vi "Set Capillary Valve.vi"(8 "error in (no error)":errorcluster, 9 "Interlock Chain.lvclass":refnum<class "Interlock Chain.lvclass">, 10 "Open? (False)":bool, 11 "Capillary Line in":refnum<class "Capillary Line.lvclass">) -> (0 "error out":errorcluster, 3 "Capillary Line out":refnum<class "Capillary Line.lvclass">)   [LabVIEW 2015, in "cRIO-Carbondioxide.lvlib" / "CO2-Actor.lvlib" / "Capillary Line.lvclass"]
uses:
  Capillary Line.lvclass
  Interlocks/Interlock Chain/Interlock Chain.lvclass
  <vilib>/ActorFramework/Actor/Actor.lvclass/Actor.ctl
  <vilib>/ActorFramework/Message Enqueuer/Message Enqueuer.lvclass/Message Enqueuer.ctl
  Capillary Line.lvclass/Capillary Line.ctl
  Valve Messages/Write Bit Field Msg/Write Bit Field Msg.lvclass/Write Bit Field Msg.ctl
  <vilib>/ActorFramework/Actor/Read Self Enqueuer.vi
  <vilib>/ActorFramework/Message Enqueuer/Enqueue.vi
  <vilib>/ActorFramework/Message Enqueuer/Init from Existing Queue.vi
  <vilib>/ActorFramework/Message Priority Queue/Priority Enqueue.vi
  <vilib>/ActorFramework/Actor/Actor.lvclass
  <vilib>/ActorFramework/Message Enqueuer/Message Enqueuer.lvclass
  Valve Messages/Write Bit Field Msg/Write Bit Field Msg.lvclass
  CO2 Actor/CO2 Actor.lvclass
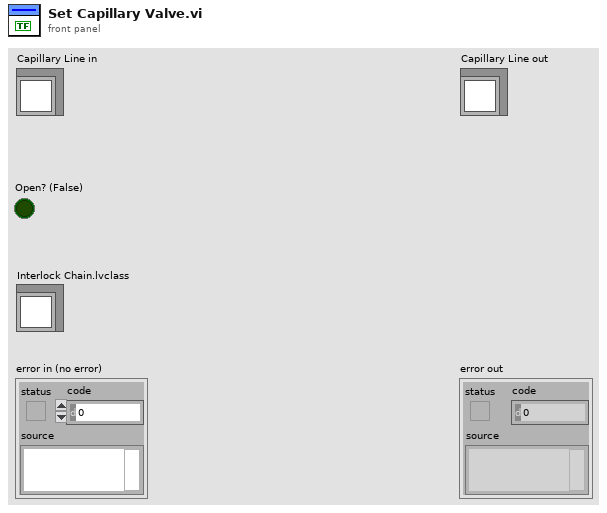
[diagram p1: front panel]
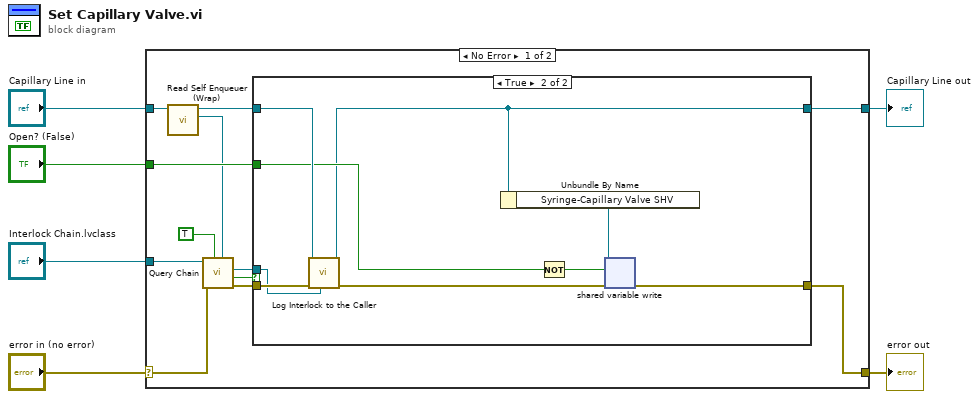
[diagram p0: block diagram]
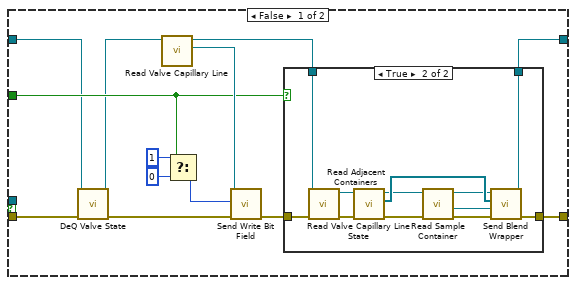
[diagram p2: hidden frame]
diagram:
  n1 = case shown="No Error" "error in (no error)" {
    selector: "error in (no error)" -> [w11 w56]
    tunnel: [w10 w56] -> w5
    tunnel: [w14 w55] -> w3
    tunnel: "Capillary Line in" -> [w9 w55]
    tunnel: "Interlock Chain.lvclass" -> [w18 _]
    tunnel: "Open? (False)" -> [w12 _]
    frame No Error {
      n2 = call "Read Self Enqueuer (Wrap).vi"("CO2 Actor in"=w9) -> ("Actor Framework:Message Enqueuer"=w7:refnum<class "Message Enqueuer.lvclass">, "CO2 Actor out"=w8:refnum<class "Capillary Line.lvclass">)  [unwired: 9 in]
      n3 = call "Query Chain.vi"("Caller Enqueuer"=w7, "Close Connections (F)"=TRUE, "error in (no error)"=w11, "Interlock Chain"=w18) -> ("error out"=w16:errorcluster, "Interlock?"=w13:bool, "Interlock out"=w15:refnum<class "Interlock.lvclass">)  [unwired: 2 in, 3 out]
      n4 = case shown="True" w13 {
        tunnel: w16 -> [w22 w54]
        tunnel: w15 -> [_ w53]
        tunnel: w8 -> [w20 w52]
        tunnel: [w28 w46] -> w14
        tunnel: w12 -> [w26 w49]
        tunnel: [w27 w47] -> w10
        frame False {
          n5 = call "DeQ Valve State.vi"("error in (no error)"=w22, "Capillary Line in"=w20) -> ("error out"=w21:errorcluster, "Capillary Line out"=w19:refnum<class "Capillary Line.lvclass">)  [unwired: 8 in]
          n6 = call "Read Valve Capillary Line.vi"("Capillary Line in"=w19) -> ("Actor Framework:Message Enqueuer"=w29:refnum<class "Message Enqueuer.lvclass">, "Capillary Line out"=w25:refnum<class "Capillary Line.lvclass">)  [unwired: 9 in]
          n7 = Select(t=u16 1, s=w26, f=u16 0 ("Bit Field")) -> (s? t:f=w23:u16)
          n8 = call "Send Write Bit Field.vi"("error in (no error)"=w21, "Bit Field"=w23, "Message Enqueuer"=w29) -> ("error out"=w24:errorcluster)  [unwired: 5 in, 3 out]
          n9 = case shown="True" w26 {
            tunnel: w24 -> [w32 w37]
            tunnel: w25 -> [w33 w35]
            tunnel: [w33 w39] -> w28
            tunnel: [w32 w38] -> w27
            frame False {
            }
            frame True {
              n10 = call "Read Valve Capillary Line State.vi"("error in (no error)"=w37, "Capillary Line in"=w35) -> ("error out"=w36:errorcluster, "Capillary Line out"=w34:refnum<class "Capillary Line.lvclass">)  [unwired: 5 in, 3 out]
              n11 = call "Read Adjacent Containers.vi"("error in (no error)"=w36, "Capillary Line in"=w34) -> ("error out"=w45:errorcluster, "Adjacent Containers"=w42:refnum<class "Message Enqueuer.lvclass">[], "Capillary Line out"=w41:refnum<class "Capillary Line.lvclass">)  [unwired: 7 in]
              n12 = call "Read Sample Container.vi"("error in (no error)"=w45, "Capillary Line in"=w41) -> ("error out"=w44:errorcluster, "Sample"=w43:refnum<class "Sample.lvclass">, "Capillary Line out"=w40:refnum<class "Capillary Line.lvclass">)  [unwired: 6 in, 1 out]
              n13 = call-dynamic "Send Blend Wrapper.vi"("error in (no error)"=w44, "Sample to Blend"=w43, "Send to"=w42, "CO2 Actor in"=w40) -> ("error out"=w38:errorcluster, "CO2 Actor out"=w39:refnum<class "Capillary Line.lvclass">)  [unwired: 6 in]
            }
          }
        }
        frame True {
          n14 = call-dynamic "Log Interlock to the Caller.vi"("Interlock in"=w53, "error in (no error)"=w54, "CO2 Actor in"=w52) -> ("error out"=w51:errorcluster, "CO2 Actor out"=w46:refnum<class "Capillary Line.lvclass">)  [unwired: 7 in]
          n15 = Unbundle By Name(w46) -> ("Syringe-Capillary Valve SHV"=w50:refnum<k21>)
          n16 = Not(x=w49) -> (.not. x?=w48:bool)
          n17 = shared-variable-write(w50, w51, w48) -> (w47:errorcluster)  [unwired: 1 out]
        }
      }
    }
    frame Error {
    }
  }
  "error out" <- w5
  "Capillary Line out" <- w3
